vi "RPT_TestInfo.vi"(8 "error in (no error)":errorcluster, 9 "Test Info":T1={"Job Number"="", "Unit Number"="", "Serial Number"="", "Technician Name"="", "Calibration Date"="", "Calibrator"="", "Calibration Slope"="", "Calibration Offset"="", "Config File Name"="Cal Date", "Notes"="Cal Date"}, 10 "font":T2 {"font size" format="%0.2f"; "strike through" items=["Strk Unchanged", "Strk Yes", "Strk No"]; "underline" items=["Und Unchanged", "Und Yes", "Und No"]; "italic" items=["Ital Unchanged", "Ital Yes", "Ital No"]; "bold" items=["Bold Unchanged", "Bold Yes", "Bold No"]}, 11 "NI_report in":refnum<class "NI_report.lvclass">) -> (0 "error out":errorcluster, 3 "NI_report out":refnum<class "NI_report.lvclass">)   [LabVIEW 2024]
uses:
  <vilib>/addons/_office/_exclsub.llb/font.ctl
  <vilib>/Utility/NIReport.llb/NI_report.lvclass
  Control Definitions/DEF_TestInfo.ctl
  <vilib>/addons/_office/NI_ReportGenerationToolkit.lvlib
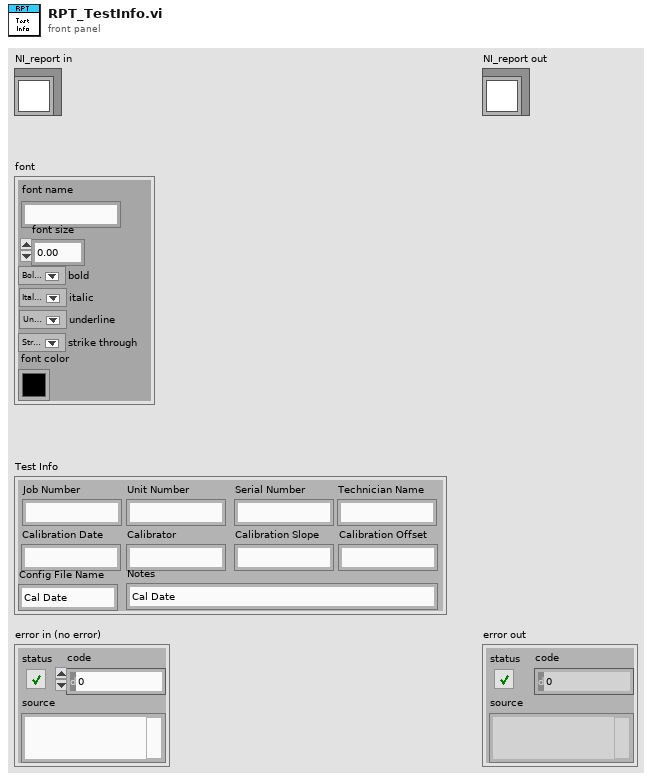
[diagram p1: front panel]
types:
  T1 = typedef "DEF_TestInfo.ctl" = cluster{"Job Number":string, "Unit Number":string, "Serial Number":string, "Technician Name":string, "Calibration Date":string, "Calibrator":string, "Calibration Slope":string, "Calibration Offset":string, "Config File Name":string, "Notes":string}
  T2 = typedef "NI_ReportGenerationToolkit.lvlib/font.ctl" = cluster{"font name":string, "font size":dbl, "bold":u16, "italic":u16, "underline":u16, "strike through":u16, "font color":u32}
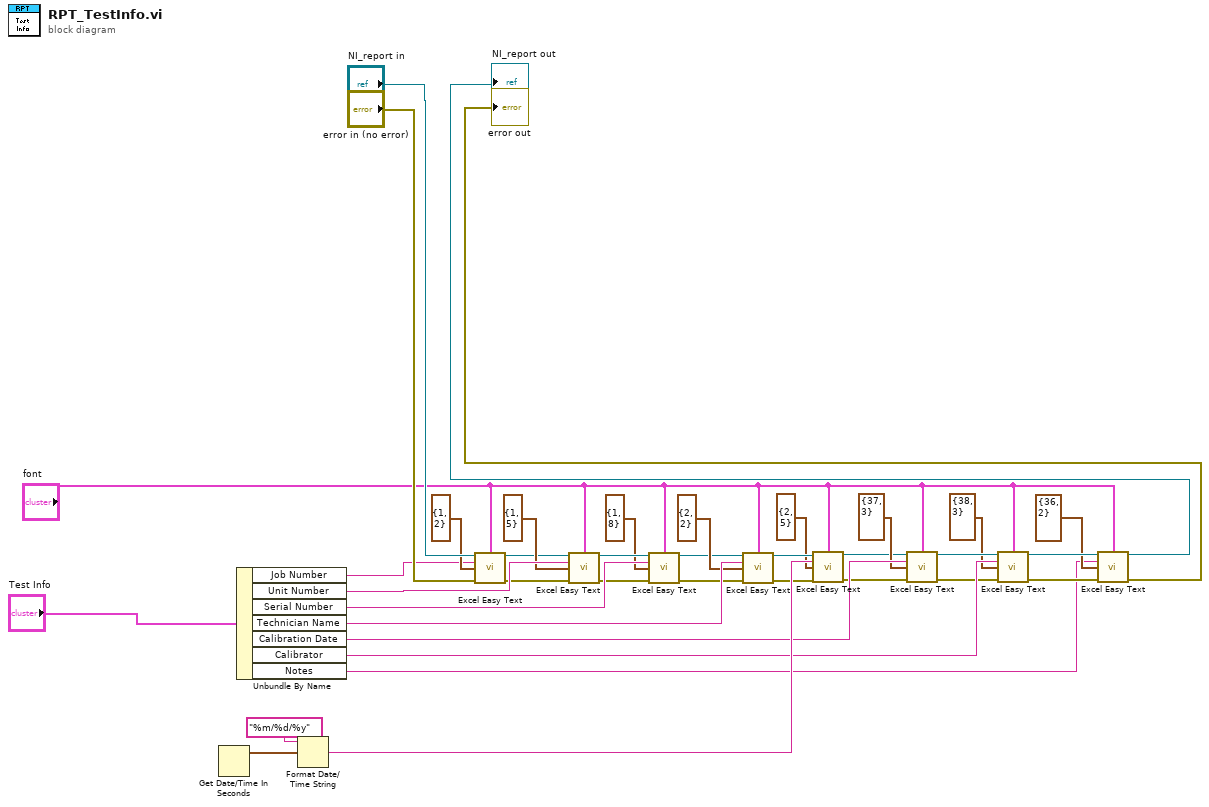
[diagram p0: block diagram]
diagram:
  n1 = Get Date/Time In Seconds() -> (seconds since 1Jan1904=w37:timestamp)
  n2 = Unbundle By Name("Test Info") -> ("Job Number"=w9:string, "Unit Number"=w22:string, "Serial Number"=w23:string, "Technician Name"=w24:string, "Calibration Date"=w35:string, "Calibrator"=w34:string, "Notes"=w1:string)
  n3 = Format Date/Time String(time format string (%c)="%m/%d/%y", seconds (now)=w37) -> (date/time string=w38:string)  [unwired: 1 in]
  n4 = call <vilib>:"Excel Easy Text.vi"("report in"="NI_report in", "font"="font", "text"=w9, "start (-1, -1)"=cluster{"row":i32, "column":i32} {"row"=1, "column"=2}, "error in (no error)"="error in (no error)") -> ("report out"=w13:refnum<class "NI_report.lvclass">, "error out"=w14:errorcluster)  [unwired: 6 in, 3 out]
  n5 = call <vilib>:"Excel Easy Text.vi"("report in"=w13, "font"="font", "text"=w22, "start (-1, -1)"=cluster{"row":i32, "column":i32} {"row"=1, "column"=5}, "error in (no error)"=w14) -> ("report out"=w20:refnum<class "NI_report.lvclass">, "error out"=w21:errorcluster)  [unwired: 6 in, 3 out]
  n6 = call <vilib>:"Excel Easy Text.vi"("report in"=w20, "font"="font", "text"=w23, "start (-1, -1)"=cluster{"row":i32, "column":i32} {"row"=1, "column"=8}, "error in (no error)"=w21) -> ("report out"=w17:refnum<class "NI_report.lvclass">, "error out"=w18:errorcluster)  [unwired: 6 in, 3 out]
  n7 = call <vilib>:"Excel Easy Text.vi"("report in"=w17, "font"="font", "text"=w24, "start (-1, -1)"=cluster{"row":i32, "column":i32} {"row"=2, "column"=2}, "error in (no error)"=w18) -> ("report out"=w30:refnum<class "NI_report.lvclass">, "error out"=w29:errorcluster)  [unwired: 6 in, 3 out]
  n8 = call <vilib>:"Excel Easy Text.vi"("report in"=w30, "font"="font", "text"=w38, "start (-1, -1)"=cluster{"row":i32, "column":i32} {"row"=2, "column"=5}, "error in (no error)"=w29) -> ("report out"=w26:refnum<class "NI_report.lvclass">, "error out"=w27:errorcluster)  [unwired: 6 in, 3 out]
  n9 = call <vilib>:"Excel Easy Text.vi"("report in"=w26, "font"="font", "text"=w35, "start (-1, -1)"=cluster{"row":i32, "column":i32} {"row"=37, "column"=3}, "error in (no error)"=w27) -> ("report out"=w33:refnum<class "NI_report.lvclass">, "error out"=w32:errorcluster)  [unwired: 6 in, 3 out]
  n10 = call <vilib>:"Excel Easy Text.vi"("report in"=w33, "font"="font", "text"=w34, "start (-1, -1)"=cluster{"row":i32, "column":i32} {"row"=38, "column"=3}, "error in (no error)"=w32) -> ("report out"=w7:refnum<class "NI_report.lvclass">, "error out"=w6:errorcluster)  [unwired: 6 in, 3 out]
  n11 = call <vilib>:"Excel Easy Text.vi"("report in"=w7, "font"="font", "text"=w1, "start (-1, -1)"=cluster{"row":i32, "column":i32} {"row"=36, "column"=2}, "error in (no error)"=w6) -> ("report out"=→"NI_report out":refnum<class "NI_report.lvclass">, "error out"=→"error out":errorcluster)  [unwired: 6 in, 3 out]
